vi "update states from tdms.vi"(8 "error in (no error)":errorcluster, 10 "frot panel referances":T1, 11 "USRP_1_x_200MHz in":refnum<class "USRP_1_x_200MHz.lvclass">) -> (0 "error out":errorcluster, 2 "tdms file mode":T2=enum."P2P - VST", 3 "USRP_1_x_200MHz out":refnum<class "USRP_1_x_200MHz.lvclass">)   [LabVIEW 2021, in "USRP_1_x_200MHz.lvclass"]
uses:
  USRP_1_x_200MHz.lvclass
  pulse_tx_vis/CTL/device_mode.ctl
  USRP_1_x_200MHz.lvclass/USRP_1_x_200MHz.ctl
  device_type/device_type.lvclass
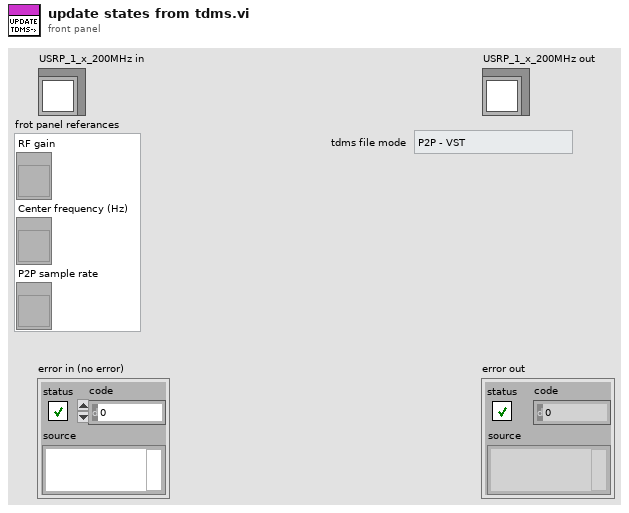
[diagram p1: front panel]
types:
  T1 = cluster{"RF gain ":refnum<vi>, "Center frequency (Hz) ":refnum<vi>, "P2P sample rate":refnum<vi>}
  T2 = typedef "device_mode.ctl" = enum16{"USRP - 180MHz", "5785 - 2*180MHz", "5785 - 3.2GHz", "P2P - VST"}
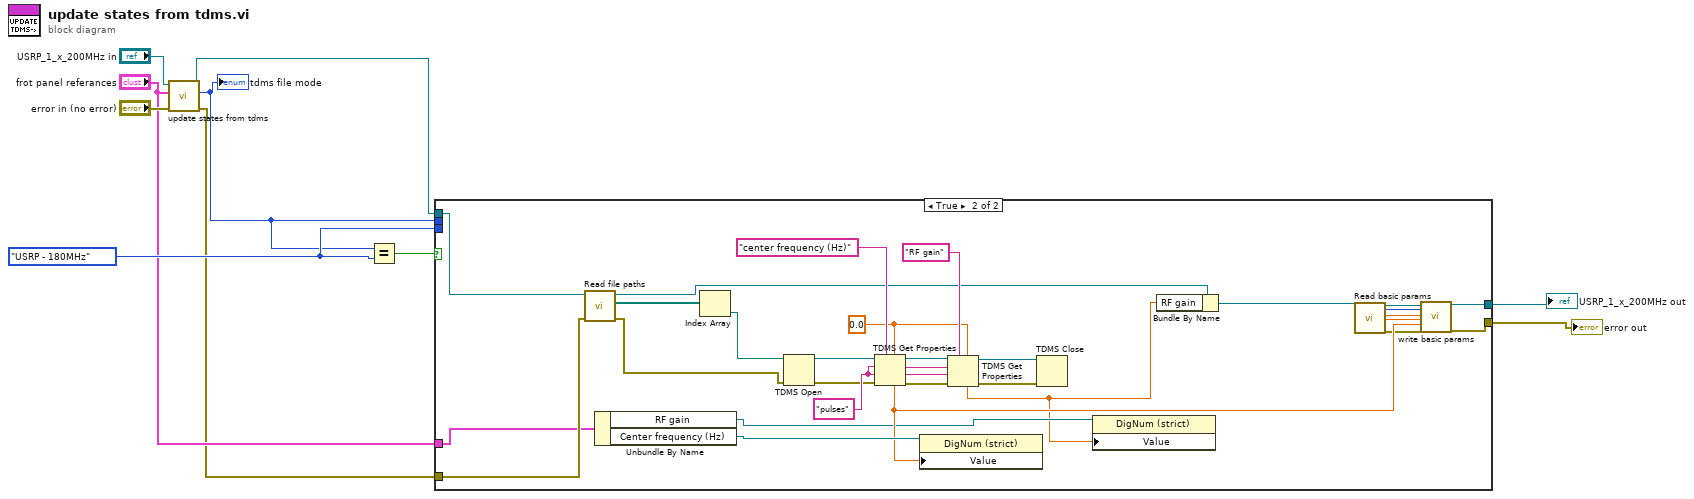
[diagram p0: block diagram]
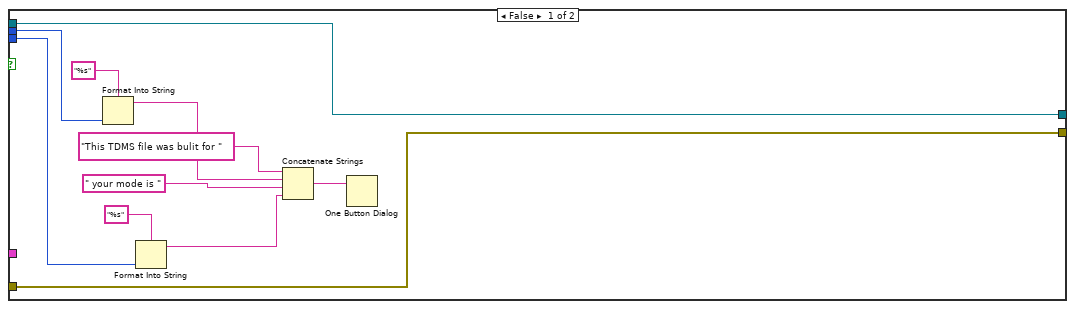
[diagram p2: hidden frame]
diagram:
  w7 = device_mode."USRP - 180MHz" ("Mode")
  n1 = call-parent "update states from tdms.vi"("error in (no error)"="error in (no error)", "frot panel referances"="frot panel referances", "device_type in"="USRP_1_x_200MHz in") -> ("error out"=w4:errorcluster, "tdms file mode"=w5:T2, "device_type out"=w3:refnum<class "USRP_1_x_200MHz.lvclass">)  [unwired: 6 in]
  "tdms file mode" <- w5
  n2 = Equal?(x=w5, y=w7) -> (x = y?=w8:bool)
  n3 = case shown="True" w8 {
    tunnel: w5 -> [w20 _]
    tunnel: w7 -> [w15 _]
    tunnel: w4 -> [w11 w47]
    tunnel: w3 -> [w12 w45]
    tunnel: "frot panel referances" -> [_ w43]
    tunnel: [w12 w35] -> w2
    tunnel: [w11 w34] -> w1
    frame False {
      n4 = Format Into String(format string="%s", w20) -> (resulting string=w19:string)  [unwired: 2 in, 1 out]
      n5 = Format Into String(format string="%s", w15) -> (resulting string=w14:string)  [unwired: 2 in, 1 out]
      n6 = Concatenate Strings("This TDMS file was bulit for " ("string"), w19, " your mode is " ("string"), w14) -> (w13:string)
      n7 = One Button Dialog(message=w13) -> ()  [unwired: 1 in, 1 out]
    }
    frame True {
      w28 = 0.0
      w52 = "pulses" ("channel name")
      n8 = call-dynamic "Read file paths.vi"("error in (no error)"=w47, "device_type in"=w45) -> ("error out"=w48:errorcluster, "file paths"=w46:path[], "device_type out"=w24:refnum<class "USRP_1_x_200MHz.lvclass">)  [unwired: 7 in]
      n9 = Unbundle By Name(w43) -> ("RF gain"=w27:refnum<vi>, "Center frequency (Hz)"=w42:refnum<vi>)
      n10 = Index Array(array=w46) -> (element=w49:path)  [unwired: 1 in]
      n11 = TDMS Open(8:w48, 11:w49) -> (0:w50:errorcluster, 3:w51:refnum<k34>)  [unwired: 5 in]
      n12 = TDMS Get Properties(5:w28, 7:"center frequency (Hz)", 8:w50, 9:w52, 10:w52, 11:w51) -> (0:w30:errorcluster, 1:w31:string, 2:w32:string, 3:w33:refnum<k34>, 4:w37:dbl)  [unwired: 1 out]
      n13 = property class="DigNum (strict)"(reference=w42, "Value"=w37) -> ()  [unwired: 1 in, 2 out]
      n14 = TDMS Get Properties(5:w28, 7:"RF gain", 8:w30, 9:w31, 10:w32, 11:w33) -> (0:w25:errorcluster, 3:w26:refnum<k34>, 4:w23:dbl)  [unwired: 3 out]
      n15 = TDMS Close(8:w25, 11:w26) -> ()  [unwired: 2 out]
      n16 = property class="DigNum (strict)"(reference=w27, "Value"=w23) -> ()  [unwired: 1 in, 2 out]
      n17 = Bundle By Name(cluster=w24, "RF gain"=w23) -> (w22:refnum<class "USRP_1_x_200MHz.lvclass">)
      n18 = call-dynamic "Read basic params.vi"("device_type in"=w22) -> ("device_type out"=w41:refnum<class "USRP_1_x_200MHz.lvclass">, "buffer size"=w40:u32, "Fs  FPGA"=w39:dbl, "SPC"=w38:dbl, "error out"=w36:errorcluster)  [unwired: 13 in, 1 out]
      n19 = call-dynamic "write basic params.vi"("device_type in"=w41, "buffer size"=w40, "Fs  FPGA"=w39, "SPC"=w38, "center frequency (Hz)"=w37, "error in (no error)"=w36) -> ("device_type out"=w35:refnum<class "USRP_1_x_200MHz.lvclass">, "error out"=w34:errorcluster)  [unwired: 12 in]
    }
  }
  "error out" <- w1
  "USRP_1_x_200MHz out" <- w2
